vi "getLastNewValueFromChannel.vi"(8 "error in (no error)":errorcluster, 10 "channelName":string, 11 "ScriptEventList in":refnum<class "ScriptEventList.lvclass">) -> (0 "error out":errorcluster, 2 "newValue":string, 3 "ScriptEventList out":refnum<class "ScriptEventList.lvclass">)   [LabVIEW 2011, in "Tools.lvlib" / "Scripting.lvlib" / "ScriptEventList.lvclass"]
uses:
  ScriptEventList.lvclass
  ScriptEventList.lvclass/ScriptEventList.ctl
  ScriptEvent.lvclass
  DatabaseHelpers/Database Objects/Channel/Channel.lvclass
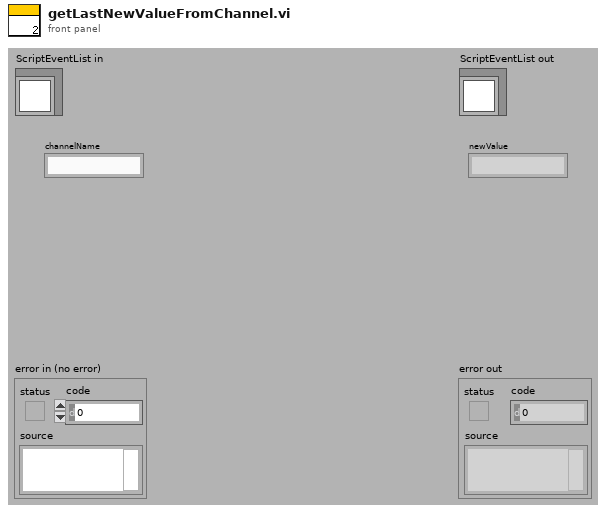
[diagram p1: front panel]
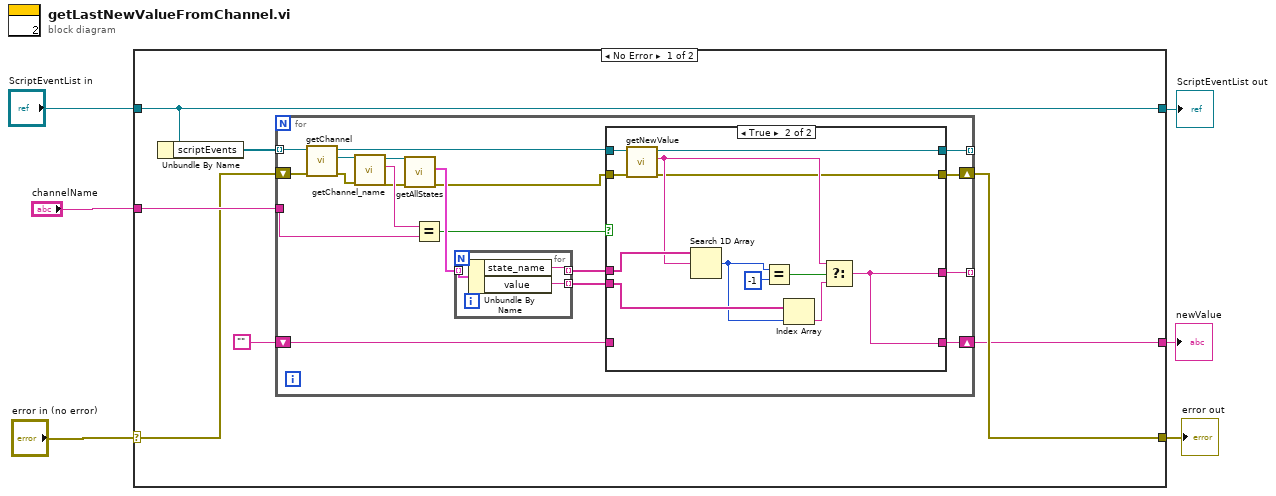
[diagram p0: block diagram]
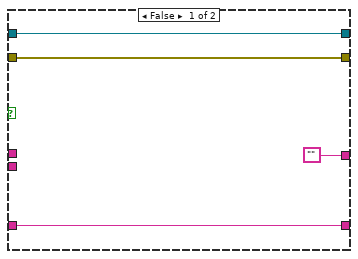
[diagram p2: hidden frame]
diagram:
  n1 = case shown="No Error" "error in (no error)" {
    selector: "error in (no error)" -> [w10 w53]
    tunnel: [w9 w53] -> w5
    tunnel: [w13 w52] -> w3
    tunnel: "ScriptEventList in" -> [w13 w52]
    tunnel: "channelName" -> [w11 _]
    tunnel: [w7 _] -> w1
    frame No Error {
      n2 = Unbundle By Name(w13) -> ("scriptEvents"=w12:refnum<class "ScriptEvent.lvclass">[])
      n3 = for {
        tunnel: w12 -> [w32] mode=indexing
        tunnel: w11 -> [w28]
        tunnel: [w20] -> _ mode=indexing
        tunnel: [w18] -> _ mode=indexing
        shift-right: [w19] -> w9
        shift-left: w10 -> [w16]
        shift-right: [w14] -> w7
        shift-left: "" -> [w15]
        n4 = call-dynamic "getChannel.vi"("error in (no error)"=w16, "ScriptEvent.lvclass in"=w32) -> ("error out"=w30:errorcluster, "Channel.lvclass"=w31:refnum<class "Channel.lvclass">, "ScriptEvent.lvclass out"=w27:refnum<class "ScriptEvent.lvclass">)  [unwired: 7 in]
        n5 = call "getChannel_name.vi"("error in (no error)"=w30, "Channel.lvclass in"=w31) -> ("error out"=w25:errorcluster, "channel_name"=w29:string, "Channel.lvclass out"=w26:refnum<class "Channel.lvclass">)  [unwired: 7 in]
        n6 = call "getAllStates.vi"("error in (no error)"=w25, "Channel.lvclass in"=w26) -> ("error out"=w23:errorcluster, "states"=w24:cluster{"state_name":string, "value":string}[])  [unwired: 7 in, 1 out]
        n7 = Equal?(x=w29, y=w28) -> (x = y?=w17:bool)
        n8 = for {
          tunnel: w24 -> [w35] mode=indexing
          tunnel: [w34] -> w21 mode=indexing
          tunnel: [w33] -> w22 mode=indexing
          n9 = Unbundle By Name(w35) -> ("state_name"=w34:string, "value"=w33:string)
        }
        n10 = case shown="True" w17 {
          tunnel: w27 -> [w38 w51]
          tunnel: w23 -> [w37 w50]
          tunnel: w21 -> [_ w49]
          tunnel: w22 -> [_ w45]
          tunnel: ["" w40] -> w18
          tunnel: [w38 w42] -> w20
          tunnel: [w37 w41] -> w19
          tunnel: w15 -> [w36 _]
          tunnel: [w36 w40] -> w14
          frame False {
          }
          frame True {
            n11 = call "getNewValue.vi"("error in (no error)"=w50, "ScriptEvent.lvclass in"=w51) -> ("error out"=w41:errorcluster, "newValue"=w46:string, "ScriptEvent.lvclass out"=w42:refnum<class "ScriptEvent.lvclass">)  [unwired: 7 in]
            n12 = Search 1D Array(1D array=w49, element=w46) -> (index of element=w44:i32)  [unwired: 1 in]
            n13 = Equal?(x=w44, y=-1) -> (x = y?=w47:bool)
            n14 = Index Array(array=w45, index=w44) -> (element=w43:string)
            n15 = Select(t=w46, s=w47, f=w43) -> (s? t:f=w40:string)
          }
        }
      }
    }
    frame Error {
    }
  }
  "error out" <- w5
  "ScriptEventList out" <- w3
  "newValue" <- w1
